vi "RT Main.vi"() -> ()   [LabVIEW 2023]
uses:
  <vilib>/Platform/TimedLoop/XDataNode/wakeup.ctl
  <vilib>/Platform/TimedLoop/XDataNode/XDNodeRunTimeDep.lvlib
  <vilib>/Platform/TimedLoop/XDataNode/nitl_modes.ctl
  <vilib>/Platform/TimedLoop/XDataNode/timing_clust.ctl
  <vilib>/platform/TimedLoop/XDataNode/XDataNode.xnode
panel:
  out "Notifiers Created":string[](array[string])
  in  "error in (no error)":errorcluster
  out "error out":errorcluster
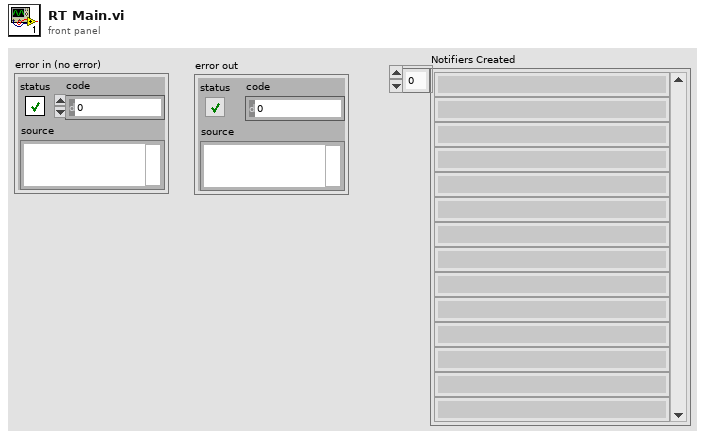
[diagram p1: front panel]
types:
  T1 = typedef "XDNodeRunTimeDep.lvlib/timing_clust.ctl" = cluster{"Expected End [f-1]":u64, "Actual End [f-1]":u64, "Finished Late? [f-1]":bool, "Expected End [i-1]":u64, "Actual End [i-1]":u64, "Finished Late? [i-1]":bool, "Expected Start [i]":u64, "Actual Start [i]":u64, "Expected Start [f]":u64, "Actual Start [f]":u64, "Source Name":string, "Structure Name":string, "Period":i64, "Deadline":i64, "Offset":i64, "Start":i64, "Priority":i32, "Timeout":i32, "Mode":T2, "Wakeup Reason":T3, "Error":errorcluster, "Source Type":string, "Secondary Source Type":string, "Global End Time":u64, "Global Start Time":u64, "Frame Duration":u64, "Iteration Duration":u64, "Assigned CPU":i32, "I/O Scan Engine Mode":u32}
  T2 = typedef "XDNodeRunTimeDep.lvlib/nitl_modes.ctl" = enum32{"No Change", "Process missed periods, maintain original phase", "Discard missed periods, maintain original phase", "Process missed periods, ignore original phase", "Discard missed periods, ignore original phase"}
  T3 = typedef "XDNodeRunTimeDep.lvlib/wakeup.ctl" = enum32{"Normal", "Aborted", "Asynchronous wakeup", "Timing source error", "Timed loop error", "Timeout"}
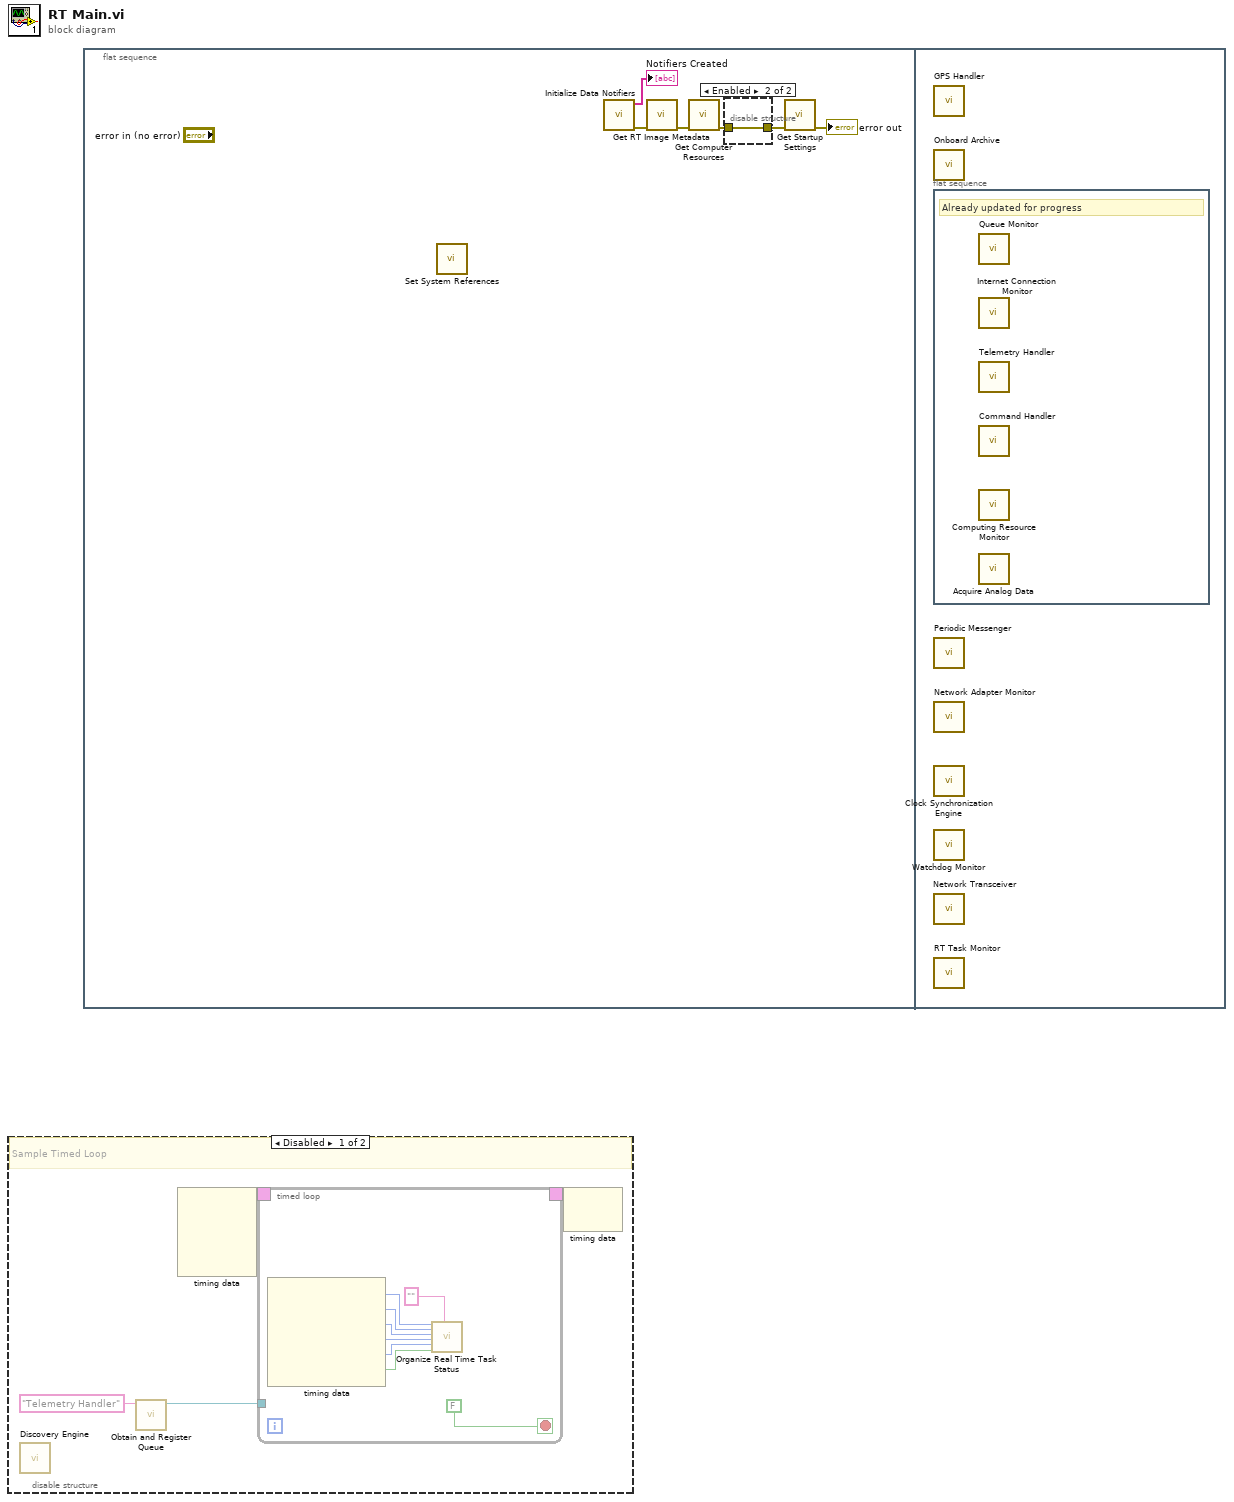
[diagram p0: block diagram]
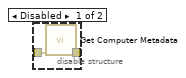
[diagram p2: hidden frame]
diagram:
  n1 = disable-structure shown="Disabled" {
    frame Disabled {
      # "Sample Timed Loop"
      n2 = call "Discovery Engine.vi"() -> ()  [unwired: 12 in]
      n3 = call "Obtain and Register Queue.vi"("Queue Name (unnamed)"="Telemetry Handler" ("name (unnamed)")) -> ("Queue Reference"=w2:refnum<queue>)  [unwired: 9 in, 1 out]
      n4 = node-c288() -> (w4:T1)  [unwired: 4 in]
      n5 = timed-loop {
        timing: w4 -> [_]
        timing-out: [_] -> w3
        tunnel: w2 -> [_]
        stop <- FALSE stop-if-true
        n6 = node-c288() -> (w10:i32, w9:i32, w8:i64, w7:i64, w6:i64, w5:bool)  [unwired: 1 in]
        n7 = call "Organize Real Time Task Status.vi"("Priority"=w10, "Processor"=w9, "Offset"=w8, "Iteration Duration"=w7, "Period"=w6, "Finished Late? [i-1]"=w5, "Task Name"="") -> ()  [unwired: 12 in, 1 out]
      }
      n8 = node-c288(w3) -> ()  [unwired: 1 out]
    }
    frame Enabled {
    }
  }
  n9 = flat-sequence {
    frame #0 {
      n10 = call "Set System References.vi"() -> ()  [unwired: 10 in, 2 out]
      n11 = call "Initialize Data Notifiers.vi"() -> ("error out"=w24:errorcluster, "Notifiers Created"=→"Notifiers Created":string[])  [unwired: 10 in]
      n12 = call "Get RT Image Metadata.vi"("error in (no error)"=w24) -> ("error out"=w25:errorcluster)  [unwired: 9 in, 1 out]
      n13 = call "Get Computer Resources.vi"("error in (no error)"=w25) -> ("error out"=w26:errorcluster)  [unwired: 9 in, 1 out]
      n14 = disable-structure shown="Enabled" {
        disable-tunnel: [w30 w31] -> w27
        disable-tunnel: w26 -> [w29 w31]
        frame Disabled {
          n15 = call "Get Computer Metadata.vi"("error in (no error)"=w29) -> ("error out"=w30:errorcluster)  [unwired: 9 in, 1 out]
        }
        frame Enabled {
        }
      }
      n16 = call "Get Startup Settings.vi"("error in (no error)"=w27) -> ("error out"=→"error out":errorcluster)  [unwired: 9 in, 1 out]
    }
    frame #1 {
      n17 = call "GPS Handler.vi"() -> ()  [unwired: 12 in]
      n18 = call "Onboard Archive.vi"() -> ()  [unwired: 12 in]
      n19 = flat-sequence {
        frame #0 {
          # "Already updated for progress"
          n20 = call "Queue Monitor.vi"() -> ()  [unwired: 12 in]
          n21 = call "Internet Connection Monitor.vi"() -> ()  [unwired: 12 in]
          n22 = call "Telemetry Handler.vi"() -> ()  [unwired: 12 in]
          n23 = call "Command Handler.vi"() -> ()  [unwired: 12 in]
          n24 = call "Computing Resource Monitor.vi"() -> ()  [unwired: 11 in, 1 out]
          n25 = call "Acquire Analog Data.vi"() -> ()  [unwired: 12 in]
        }
      }
      n26 = call "Periodic Messenger.vi"() -> ()  [unwired: 12 in]
      n27 = call "Network Adapter Monitor.vi"() -> ()  [unwired: 12 in]
      n28 = call "Clock Synchronization Engine.vi"() -> ()  [unwired: 12 in]
      n29 = call "Watchdog Monitor.vi"() -> ()  [unwired: 12 in]
      n30 = call "Network Transceiver.vi"() -> ()  [unwired: 12 in]
      n31 = call "RT Task Monitor.vi"() -> ()  [unwired: 12 in]
    }
  }
